vi "sv_Check for Frequency Change [Full Octave].vi"(7 "reset filter (F)":bool, 8 "error in (no error)":errorcluster, 9 "frequency range (1/1)":T1={"low band"=enum."16 Hz", "high band"=enum."16000 Hz"}) -> (0 "error out":errorcluster, 2 "Param_has_changed":bool)   [LabVIEW 2017, in "SoundVib_Octave_2014 standard.lvlib"]
uses:
  <vilib>/addons/Sound and Vibration/svt_Octave/SoundVib_Octave_2014 standard.lvlib
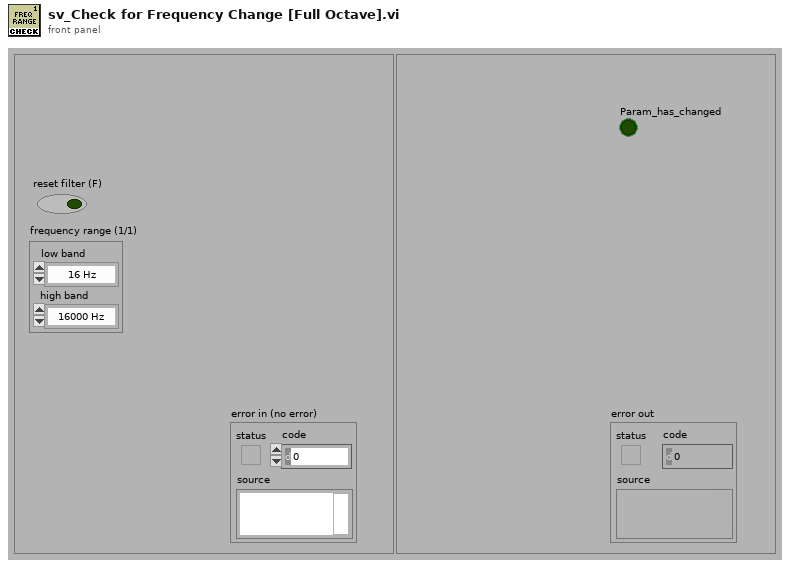
[diagram p1: front panel]
types:
  T1 = cluster{"low band":enum16{"16 Hz", "31.5 Hz", "63 Hz", "125 Hz", "250 Hz", "500 Hz", "1000 Hz", "2000 Hz", "4000 Hz", "8000 Hz", "16000 Hz"}, "high band":enum16{"16 Hz", "31.5 Hz", "63 Hz", "125 Hz", "250 Hz", "500 Hz", "1000 Hz", "2000 Hz", "4000 Hz", "8000 Hz", "16000 Hz"}}
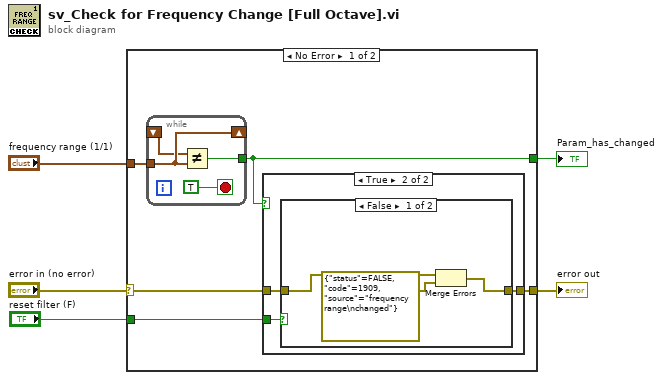
[diagram p0: block diagram]
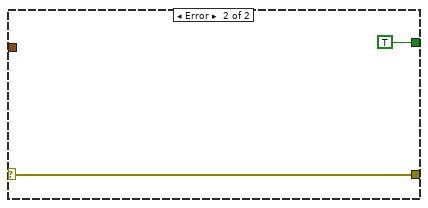
[diagram p4: hidden frame]
diagram:
  n1 = case shown="No Error" "error in (no error)" {
    selector: "error in (no error)" -> [w7 w24]
    tunnel: "frequency range (1/1)" -> [w10 _]
    tunnel: [w9 TRUE] -> w4
    tunnel: [w8 w24] -> w3
    tunnel: "reset filter (F)" -> [w6 _]
    frame No Error {
      n2 = while {
        tunnel: w10 -> [w12]
        tunnel: [w13] -> w9
        shift-left: _ -> [w11]
        shift-right: [w12] -> _
        stop <- TRUE stop-if-true
        n3 = Not Equal?(x=w11, y=w12) -> (x != y?=w13:bool)
      }
      n4 = case shown="True" w9 {
        tunnel: w7 -> [w15 w16]
        tunnel: [w15 w18] -> w8
        tunnel: w6 -> [_ w17]
        frame False {
        }
        frame True {
          n5 = case shown="False" w17 {
            tunnel: [w20 w22] -> w18
            tunnel: w16 -> [w19 w22]
            frame False {
              n6 = Merge Errors(w19, errorcluster {"status"=FALSE, "code"=1909, "source"="frequency range\nchanged"} ("error IO")) -> (w20:errorcluster)
            }
            frame True {
            }
          }
        }
      }
    }
    frame Error {
    }
  }
  "error out" <- w3
  "Param_has_changed" <- w4
